vi "QuickShoot.vi"() -> ()   [LabVIEW 2012]
uses:
  State_Machine_Enum.ctl
  Sally_Dashboard_2014/DBNameEnum.ctl
  Robot Global Data.vi
panel:
  in  "PullBackTolerenceMaxPercentDifference":dbl=0.1
  in  "FireTolerenceRPM 2":dbl=5.0
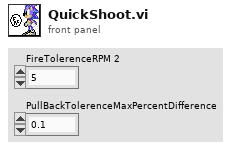
[diagram p1: front panel]
types:
  T1 = typedef "State_Machine_Enum.ctl" = enum16{"Idle", "Start", "Do", "Stop", "Init"}
  T2 = typedef "DBNameEnum.ctl" = enum16{"AutoInstructions", "DriveLoopTime", "DriveAlignLSLeft", "DriveAlignLSRight", "Use2DriveAlign", "ClimbLS", "LauncherAngleMatches", "FrameworkVersion", "sLauncherAngle", "LauncherTargetAngle", "sLauncherRPM", "LauncherTargetRPM", "sDriveDistance", "LauncherMotorValue", "PullbackTol", "FireTol", "LauncherRPMTol", "LauncherAngleTol", "InitialWait", "WaitBetweenLaunch", "AnglePresets", "RPMPresets", "UseAngleEncoder", "UseLauncherEncoder", "UseLauncherPID", "QSWaitBeforeFire", "QSWaitBeforeRetract", "AngleForwardValue", "AngleBackwardValue", "UseClusterArray", "BackupAuto", "ReverseDriveIndicate", "HalfSpeedFactor"}
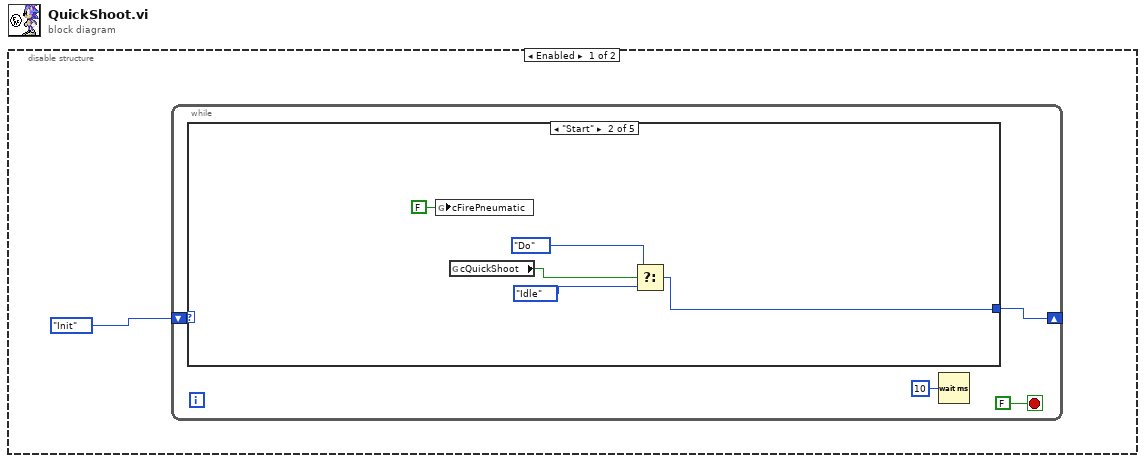
[diagram p0: block diagram]
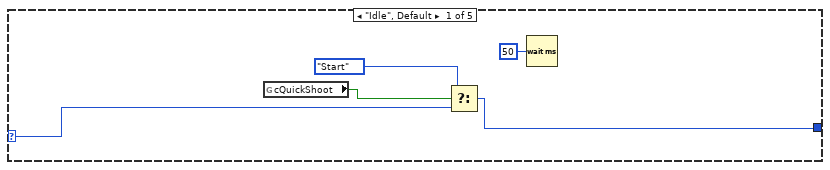
[diagram p2: hidden frame]
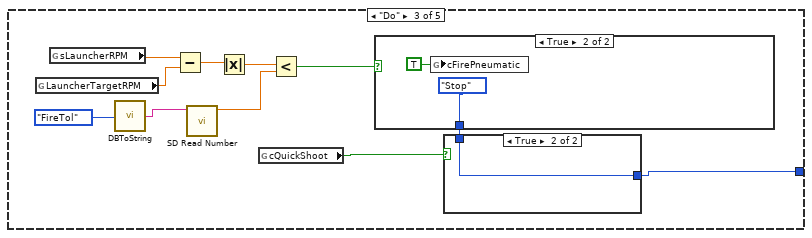
[diagram p3: hidden frame]
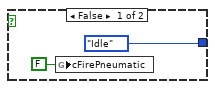
[diagram p4: hidden frame]
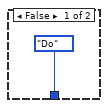
[diagram p5: hidden frame]
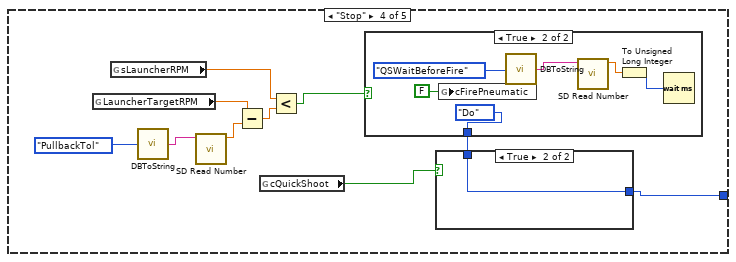
[diagram p6: hidden frame]
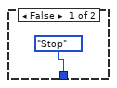
[diagram p7: hidden frame]
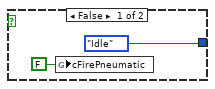
[diagram p8: hidden frame]
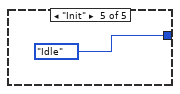
[diagram p9: hidden frame]
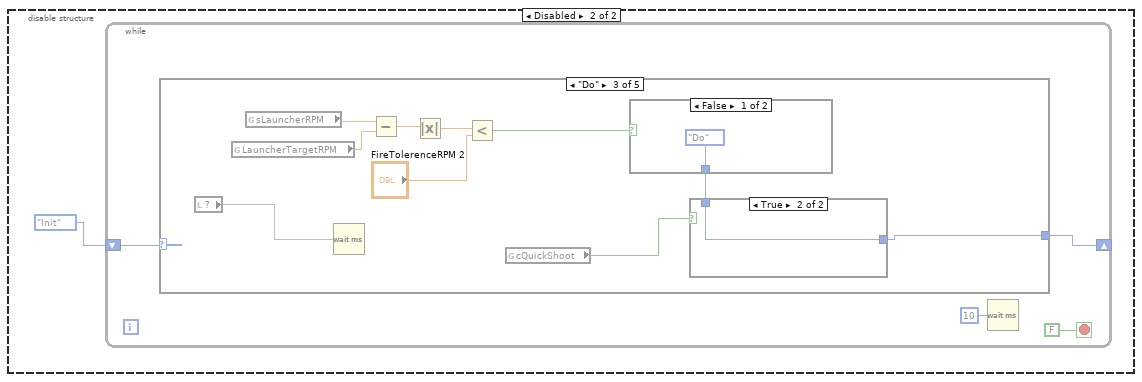
[diagram p10: hidden frame]
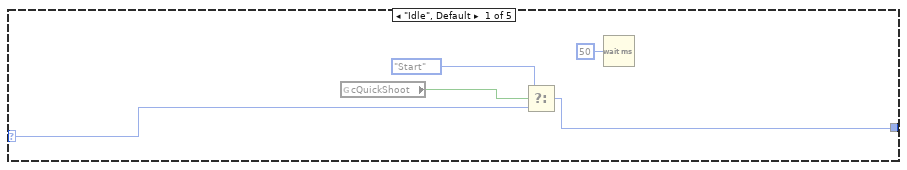
[diagram p11: hidden frame]
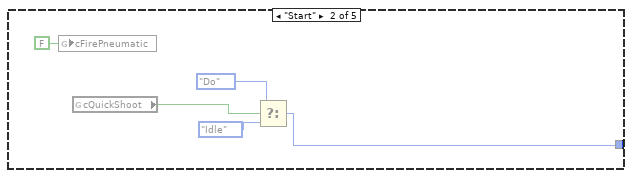
[diagram p12: hidden frame]
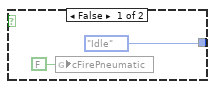
[diagram p13: hidden frame]
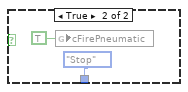
[diagram p14: hidden frame]
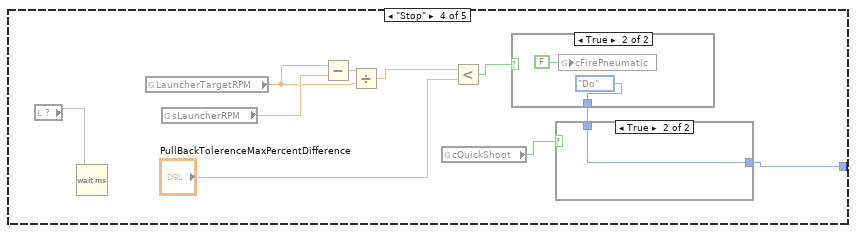
[diagram p15: hidden frame]
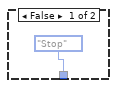
[diagram p16: hidden frame]
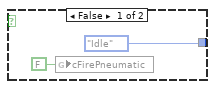
[diagram p17: hidden frame]
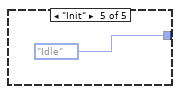
[diagram p18: hidden frame]
diagram:
  n1 = disable-structure shown="Enabled" {
    frame Enabled {
      n2 = while {
        shift-right: [w3] -> _
        shift-left: State_Machine_Enum."Init" ("State") -> [w4]
        stop <- FALSE stop-if-true
        n3 = case shown="\"Start\"" w4 {
          selector: w4 -> [w10 _ _ _ _]
          tunnel: [w9 w13 w19 w42 State_Machine_Enum."Idle" ("State")] -> w3
          frame "Idle", Default {
            n4 = global read "Robot Global Data.vi" "cQuickShoot"() -> (w8:bool)
            n5 = Select(t=State_Machine_Enum."Start", s=w8, f=w10) -> (s? t:f=w9:T1)
            n6 = Wait (ms)(milliseconds to wait=u32 50) -> ()  [unwired: 1 out]
          }
          frame "Start" {
            n7 = global write "Robot Global Data.vi" "cFirePneumatic"(FALSE ("cFirePneumatic")) -> ()
            n8 = global read "Robot Global Data.vi" "cQuickShoot"() -> (w15:bool)
            n9 = Select(t=State_Machine_Enum."Do", s=w15, f=State_Machine_Enum."Idle") -> (s? t:f=w13:T1)
          }
          frame "Do" {
            n10 = global read "Robot Global Data.vi" "LauncherTargetRPM"() -> (w25:dbl)
            n11 = global read "Robot Global Data.vi" "sLauncherRPM"() -> (w26:dbl)
            n12 = call "DBToString.vi"("Enum"=DBNameEnum."FireTol") -> ("Refname"=w16:string)
            n13 = Subtract(x=w26, y=w25) -> (x-y=w24:dbl)
            n14 = call <vilib>:"SD Read Number.vi"("Name"=w16) -> ("Numeric"=w18:dbl)  [unwired: 8 in, 2 out]
            n15 = Absolute Value(x=w24) -> (abs(x)=w23:dbl)
            n16 = global read "Robot Global Data.vi" "cQuickShoot"() -> (w21:bool)
            n17 = Less?(x=w23, y=w18) -> (x < y?=w22:bool)
            n18 = case shown="True" w22 {
              tunnel: [State_Machine_Enum."Do" ("t") State_Machine_Enum."Stop" ("t")] -> w20
              frame False {
              }
              frame True {
                n19 = global write "Robot Global Data.vi" "cFirePneumatic"(TRUE ("cFirePneumatic")) -> ()
              }
            }
            n20 = case shown="True" w21 {
              tunnel: [State_Machine_Enum."Idle" ("f") w29] -> w19
              tunnel: w20 -> [_ w29]
              frame False {
                n21 = global write "Robot Global Data.vi" "cFirePneumatic"(FALSE ("cFirePneumatic")) -> ()
              }
              frame True {
              }
            }
          }
          frame "Stop" {
            n22 = global read "Robot Global Data.vi" "LauncherTargetRPM"() -> (w40:dbl)
            n23 = global read "Robot Global Data.vi" "sLauncherRPM"() -> (w39:dbl)
            n24 = call "DBToString.vi"("Enum"=DBNameEnum."PullbackTol") -> ("Refname"=w33:string)
            n25 = call <vilib>:"SD Read Number.vi"("Name"=w33) -> ("Numeric"=w35:dbl)  [unwired: 8 in, 2 out]
            n26 = Subtract(x=w40, y=w35) -> (x-y=w38:dbl)
            n27 = global read "Robot Global Data.vi" "cQuickShoot"() -> (w41:bool)
            n28 = Less?(x=w39, y=w38) -> (x < y?=w37:bool)
            n29 = case shown="True" w37 {
              tunnel: [State_Machine_Enum."Stop" ("t") State_Machine_Enum."Do" ("t")] -> w36
              frame False {
              }
              frame True {
                n30 = global write "Robot Global Data.vi" "cFirePneumatic"(FALSE ("cFirePneumatic")) -> ()
                n31 = call "DBToString.vi"("Enum"=DBNameEnum."QSWaitBeforeFire") -> ("Refname"=w46:string)
                n32 = call <vilib>:"SD Read Number.vi"("Name"=w46) -> ("Numeric"=w45:dbl)  [unwired: 8 in, 2 out]
                n33 = To Unsigned Long Integer(number=w45) -> (unsigned 32bit integer=w44:u32)
                n34 = Wait (ms)(milliseconds to wait=w44) -> ()  [unwired: 1 out]
              }
            }
            n35 = case shown="True" w41 {
              tunnel: [State_Machine_Enum."Idle" ("f") w52] -> w42
              tunnel: w36 -> [_ w52]
              frame False {
                n36 = global write "Robot Global Data.vi" "cFirePneumatic"(FALSE ("cFirePneumatic")) -> ()
              }
              frame True {
              }
            }
          }
          frame "Init" {
          }
        }
        n37 = Wait (ms)(milliseconds to wait=u32 10) -> ()  [unwired: 1 out]
      }
    }
    frame Disabled {
      n38 = while {
        shift-right: [w56] -> _
        shift-left: State_Machine_Enum."Init" ("State") -> [w57]
        stop <- FALSE stop-if-true
        n39 = case shown="\"Do\"" w57 {
          selector: w57 -> [w63 _ _ _ _]
          tunnel: [w62 w66 w75 w94 State_Machine_Enum."Idle" ("State")] -> w56
          frame "Idle", Default {
            n40 = global read "Robot Global Data.vi" "cQuickShoot"() -> (w61:bool)
            n41 = Select(t=State_Machine_Enum."Start", s=w61, f=w63) -> (s? t:f=w62:T1)
            n42 = Wait (ms)(milliseconds to wait=u32 50) -> ()  [unwired: 1 out]
          }
          frame "Start" {
            n43 = global write "Robot Global Data.vi" "cFirePneumatic"(FALSE ("cFirePneumatic")) -> ()
            n44 = global read "Robot Global Data.vi" "cQuickShoot"() -> (w68:bool)
            n45 = Select(t=State_Machine_Enum."Do", s=w68, f=State_Machine_Enum."Idle") -> (s? t:f=w66:T1)
          }
          frame "Do" {
            n46 = local read item#-1() -> (w69)
            n47 = global read "Robot Global Data.vi" "LauncherTargetRPM"() -> (w73:dbl)
            n48 = global read "Robot Global Data.vi" "sLauncherRPM"() -> (w74:dbl)
            n49 = Wait (ms)(milliseconds to wait=w69) -> ()  [unwired: 1 out]
            n50 = Subtract(x=w74, y=w73) -> (x-y=w72:dbl)
            n51 = Absolute Value(x=w72) -> (abs(x)=w70:dbl)
            n52 = Less?(x=w70, y="FireTolerenceRPM 2") -> (x < y?=w78:bool)
            n53 = global read "Robot Global Data.vi" "cQuickShoot"() -> (w77:bool)
            n54 = case shown="False" w78 {
              tunnel: [State_Machine_Enum."Do" ("t") State_Machine_Enum."Stop" ("t")] -> w76
              frame False {
              }
              frame True {
                n55 = global write "Robot Global Data.vi" "cFirePneumatic"(TRUE ("cFirePneumatic")) -> ()
              }
            }
            n56 = case shown="True" w77 {
              tunnel: [State_Machine_Enum."Idle" ("f") w81] -> w75
              tunnel: w76 -> [_ w81]
              frame False {
                n57 = global write "Robot Global Data.vi" "cFirePneumatic"(FALSE ("cFirePneumatic")) -> ()
              }
              frame True {
              }
            }
          }
          frame "Stop" {
            n58 = local read item#-1() -> (w85)
            n59 = Wait (ms)(milliseconds to wait=w85) -> ()  [unwired: 1 out]
            n60 = global read "Robot Global Data.vi" "LauncherTargetRPM"() -> (w86:dbl)
            n61 = global read "Robot Global Data.vi" "sLauncherRPM"() -> (w88:dbl)
            n62 = Subtract(x=w86, y=w88) -> (x-y=w87:dbl)
            n63 = Divide(x=w87, y=w86) -> (x/y=w90:dbl)
            n64 = global read "Robot Global Data.vi" "cQuickShoot"() -> (w93:bool)
            n65 = Less?(x=w90, y="PullBackTolerenceMaxPercentDifference") -> (x < y?=w92:bool)
            n66 = case shown="True" w92 {
              tunnel: [State_Machine_Enum."Stop" ("t") State_Machine_Enum."Do" ("t")] -> w91
              frame False {
              }
              frame True {
                n67 = global write "Robot Global Data.vi" "cFirePneumatic"(FALSE ("cFirePneumatic")) -> ()
              }
            }
            n68 = case shown="True" w93 {
              tunnel: [State_Machine_Enum."Idle" ("f") w100] -> w94
              tunnel: w91 -> [_ w100]
              frame False {
                n69 = global write "Robot Global Data.vi" "cFirePneumatic"(FALSE ("cFirePneumatic")) -> ()
              }
              frame True {
              }
            }
          }
          frame "Init" {
          }
        }
        n70 = Wait (ms)(milliseconds to wait=u32 10) -> ()  [unwired: 1 out]
      }
    }
  }
